vi "Actor Core.vi"(8 "error in":errorcluster, 11 "Caller in":refnum<class "Caller.lvclass">) -> (0 "error out":errorcluster, 3 "Actor out":refnum<class "Actor.lvclass">)   [LabVIEW 2020, in "Caller.lvlib" / "Caller.lvclass"]
doc: "(<B>Filename</B>: Actor Framework.lvlib:Actor.lvclass:Actor Core.vi)\n\nReceives messages to the actor, reacts to them, and initiates any error handling that may shut the actor down.\n\nDescendant classes may override this VI to append parallel tasks for the actor to complete while it handles messages. Overrides use the Call Parent Class Method node."
uses:
  Caller.lvclass
  <vilib>/ActorFramework/Actor/Actor.lvclass
  Caller.lvclass/Caller.ctl
  <vilib>/ActorFramework/Message Enqueuer/Message Enqueuer.lvclass/Message Enqueuer.ctl
  Caller Messages/SendNested Msg/SendNested Msg.lvclass/SendNested Msg.ctl
  <vilib>/ActorFramework/Message Enqueuer/Enqueue.vi
  Caller Messages/LaunchNested Msg/LaunchNested Msg.lvclass
  C:/Program Files/National Instruments/LabVIEW 2020/vi.lib/ActorFramework/Message/Message.lvclass
  Caller Messages/SendNested Msg/SendNested Msg.lvclass
  <vilib>/ActorFramework/Stop Msg/Stop Msg.lvclass
  <vilib>/ActorFramework/Message Priority Queue/Priority Enqueue.vi
panel:
  out "Nested cpt ?":u8
  in  "Btn_Error":bool
  in  "Btn_Launch_Nested":bool
  in  "Message":string
  out "Display":string
  in  "Btn_ Send_Nested":bool
  # "Caller"
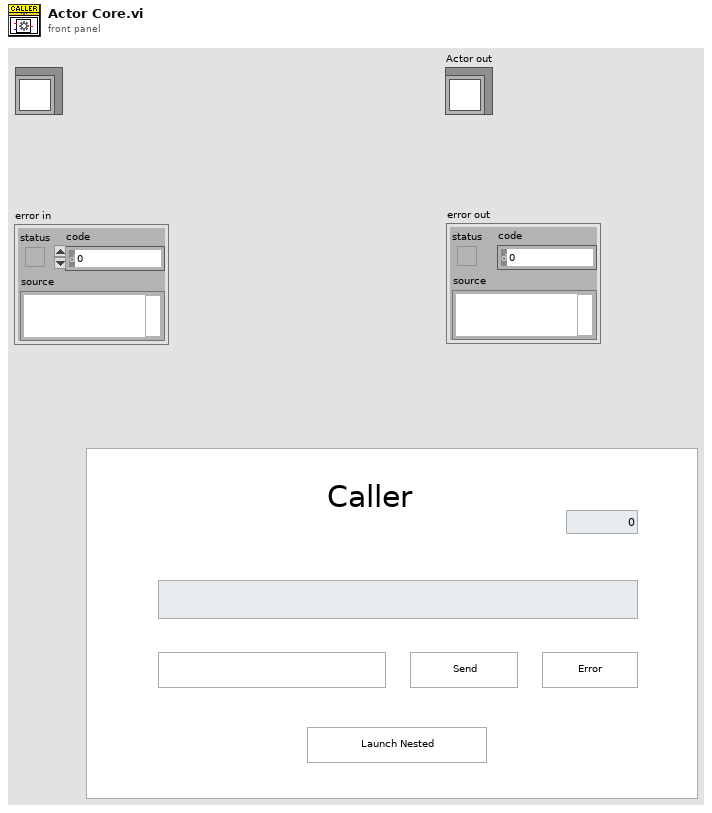
[diagram p1: front panel]
types:
  T1 = cluster{"Quit":refnum<user-event>, "Display":refnum<user-event>, "Cpt Nested":refnum<user-event>}
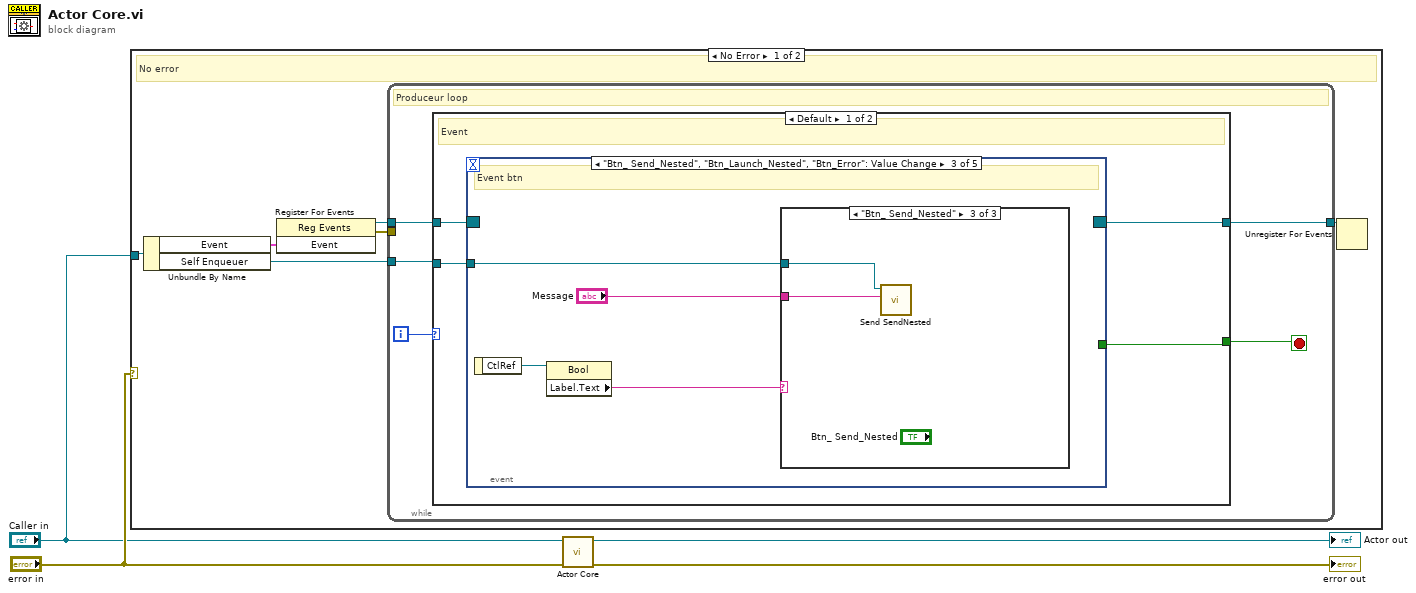
[diagram p0: block diagram]
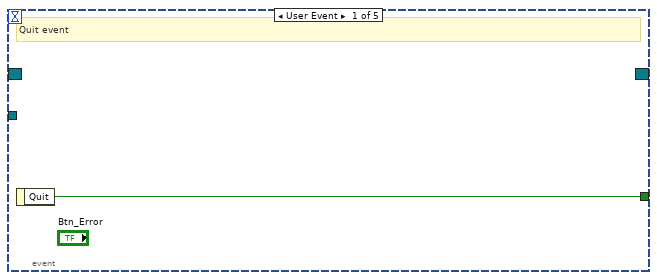
[diagram p2: hidden frame]
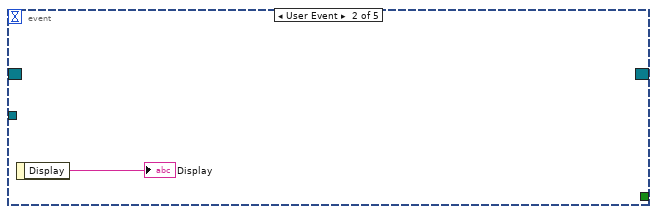
[diagram p3: hidden frame]
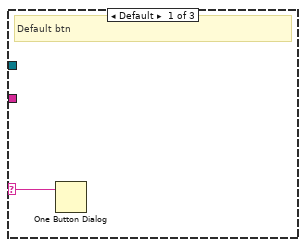
[diagram p4: hidden frame]
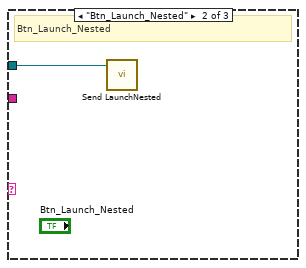
[diagram p5: hidden frame]
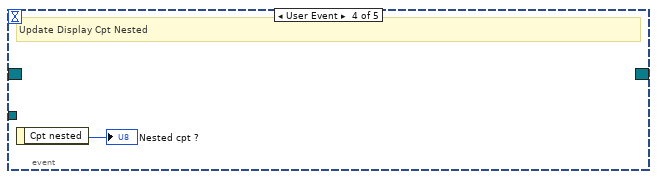
[diagram p6: hidden frame]
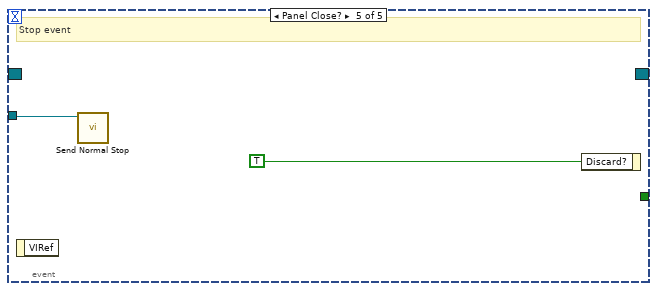
[diagram p7: hidden frame]
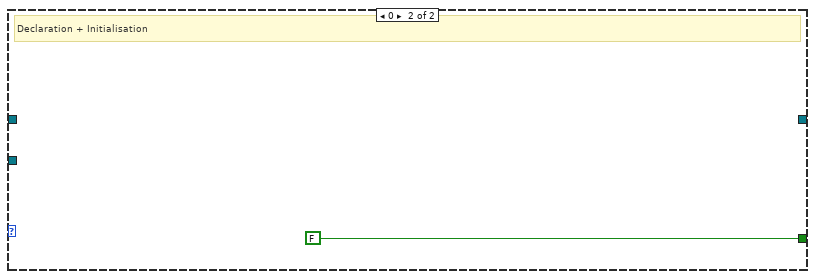
[diagram p8: hidden frame]
diagram:
  n1 = case shown="No Error" "error in" {
    tunnel: "Caller in" -> [w8 _]
    frame No Error {
      # "No error"
      n2 = Unbundle By Name(w8) -> ("Event"=w6:T1, "Self Enqueuer"=w9:refnum<class "Message Enqueuer.lvclass">)
      n3 = register-events(w6) -> (reference out=w7:refnum<event-registration>, error out=w5:errorcluster)  [unwired: 2 in]
      n4 = while {
        tunnel: [w13] -> w10
        tunnel: w9 -> [w12]
        tunnel: w7 -> [w11]
        tunnel: w5 -> [_]
        i -> [w15]
        stop <- w14 stop-if-true
        # "Produceur loop"
        n5 = case shown="Default" w15 {
          tunnel: w12 -> [w17 _]
          tunnel: [w18 FALSE] -> w14
          tunnel: [w19 _] -> w13
          tunnel: w11 -> [w16 _]
          frame Default {
            # "Event"
            n6 = event shown="[2] \"Btn_ Send_Nested\", \"Btn_Launch_Nested\", \"Btn_Error\": Value Change" {
              selector: w16 -> [_ _ _ _ _]
              dyn-events: [_ _ _ _ _] -> w19
              timeout: _ -> [_ _ _ _ _]
              tunnel: [w20 _ _ _ _] -> w18
              tunnel: w17 -> [_ _ w23 _ w31]
              event User Event {
                # "Quit event"
                n7 = event-data() -> ("Quit"=w20:bool)  [unwired: 1 in]
              }
              event User Event {
                n8 = event-data() -> ("Display"=→"Display":string)  [unwired: 1 in]
              }
              event "Btn_ Send_Nested", "Btn_Launch_Nested", "Btn_Error": Value Change {
                # "Event btn"
                n9 = event-data() -> ("CtlRef"=w25:refnum<vi>)  [unwired: 1 in]
                n10 = property class="Bool"(reference=w25) -> ("Label.Text"=w24:string)  [unwired: 1 in, 2 out]
                n11 = case shown="\"Btn_ Send_Nested\"" w24 {
                  selector: w24 -> [w26 _ _]
                  tunnel: w23 -> [_ w27 w29]
                  tunnel: "Message" -> [_ _ w28]
                  frame Default {
                    # "Default btn"
                    n12 = One Button Dialog(message=w26) -> ()  [unwired: 1 in, 1 out]
                  }
                  frame "Btn_Launch_Nested" {
                    # "Btn_Launch_Nested"
                    n13 = call "Send LaunchNested.vi"("Message Enqueuer"=w27) -> ()  [unwired: 9 in, 2 out]
                  }
                  frame "Btn_ Send_Nested" {
                    n14 = call "Send SendNested.vi"("Message"=w28, "Message Enqueuer"=w29) -> ()  [unwired: 8 in, 2 out]
                  }
                }
              }
              event User Event {
                # "Update Display Cpt Nested"
                n15 = event-data() -> ("Cpt nested"=→"Nested cpt ?":u8)  [unwired: 1 in]
              }
              event Panel Close? {
                # "Stop event"
                n16 = event-data() -> ()  [unwired: 1 in, 1 out]
                n17 = call <vilib>:"Send Normal Stop.vi"("Message Enqueuer"=w31) -> ()  [unwired: 10 in, 1 out]
                n18 = event-data("Discard?"=TRUE) -> ()  [unwired: 1 in, 1 out]
              }
            }
          }
          frame 0 {
            # "Declaration + Initialisation"
          }
        }
      }
      n19 = Unregister For Events(event registration refnum=w10) -> ()  [unwired: 1 in, 1 out]
    }
    frame Error {
    }
  }
  n20 = call-parent "Actor Core.vi"("error in"="error in", "Actor in"="Caller in") -> ("error out"=→"error out":errorcluster, "Actor out"=→"Actor out":refnum<class "Actor.lvclass">)  [unwired: 8 in]
